vi "ArduinoRead.vi"(0 "VISA resource name":refnum<visa-resource-name>="COM24", 5 "Arduino function":enum16{"Interlock", "Edgesense", "Humidity"}(ring), 7 "Humidity IN":dbl[](array[numeric]), 9 "Temperature IN":dbl[](array[numeric]), 11 "error in (no error)":errorcluster) -> (2 "VISA resource name OUT":refnum<visa-resource-name>="COM24", 3 "Edgesense Status":u16(ring)=1 items=["Contact", "No contact"], 4 "Temperature [°C]":dbl, 6 "rel. Humidity [%]":dbl, 8 "Humidity OUT":dbl[](array[numeric]), 10 "Temperature OUT":dbl[](array[numeric]), 14 "error out":errorcluster, 15 "Interlock Status":u16(ring) items=["Dark", "Light"])   [LabVIEW 2013, in "ArduinoControl.lvclass"]
uses:
  ArduinoControl.lvclass
panel:
  out "String":string
  out "return count":u32
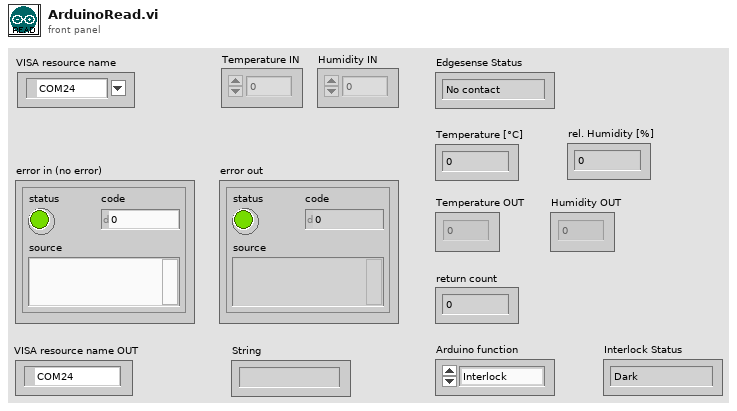
[diagram p1: front panel]
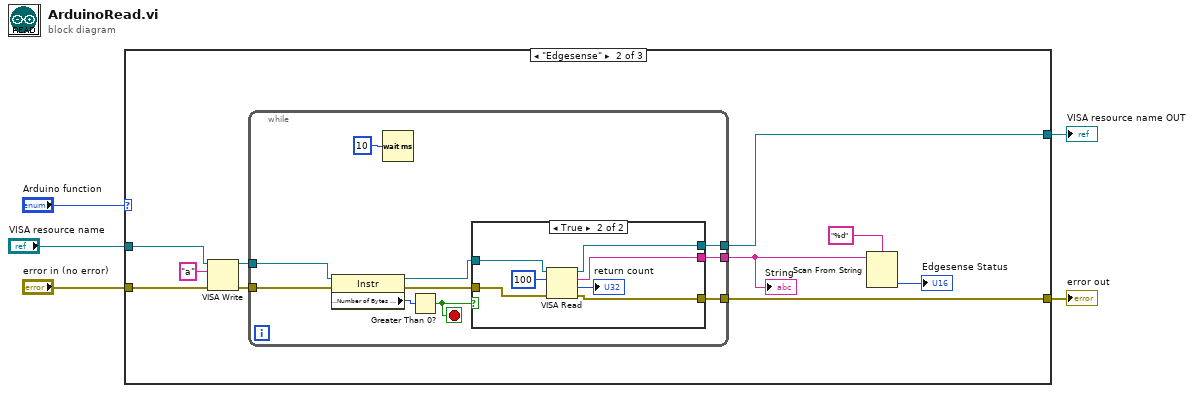
[diagram p0: block diagram]
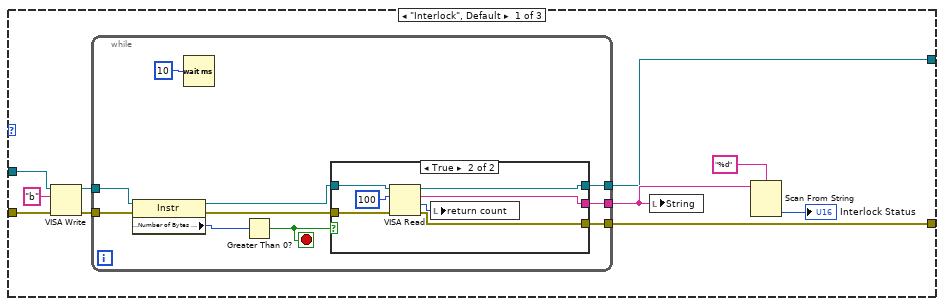
[diagram p2: hidden frame]
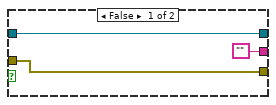
[diagram p3: hidden frame]
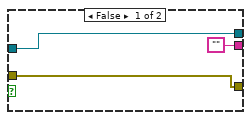
[diagram p4: hidden frame]
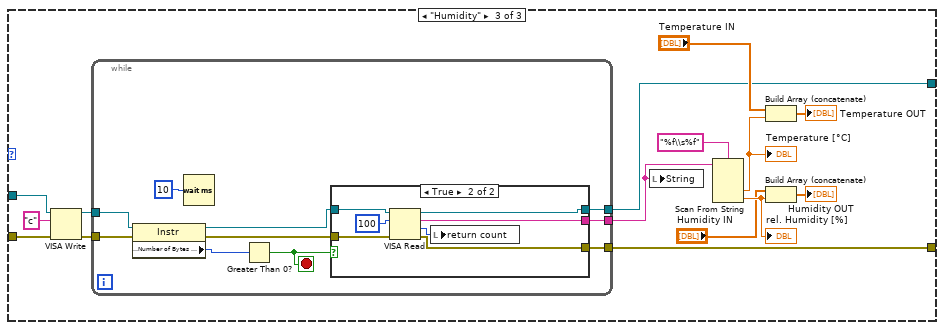
[diagram p5: hidden frame]
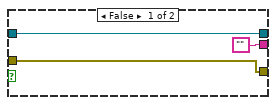
[diagram p6: hidden frame]
diagram:
  n1 = case shown="\"Edgesense\"" "Arduino function" {
    tunnel: "error in (no error)" -> [w7 w38 w68]
    tunnel: "VISA resource name" -> [w9 w39 w70]
    tunnel: [w12 w41 w71] -> w5
    tunnel: [w11 w42 w72] -> w4
    frame "Interlock", Default {
      n2 = VISA Write(VISA resource name=w9, write buffer="b", error in (no error)=w7) -> (VISA resource name out=w8:refnum<visa-resource-name>, error out=w6:errorcluster)  [unwired: 1 out]
      n3 = while {
        tunnel: [w23] -> w12
        tunnel: [w22] -> w13
        tunnel: w6 -> [w16]
        tunnel: w8 -> [w17]
        tunnel: [w21] -> w11
        stop <- w18 stop-if-true
        n4 = property class="Instr"(reference=w17, error in=w16) -> (reference out=w25:refnum<visa-resource-name>, error out=w24:errorcluster, "Serial Settings:Number of Bytes at Serial Port"=w19:u32)
        n5 = Wait (ms)(milliseconds to wait=10) -> ()  [unwired: 1 out]
        n6 = Greater Than 0?(x=w19) -> (x > 0?=w18:bool)
        n7 = case shown="True" w18 {
          tunnel: w25 -> [w26 w35]
          tunnel: w24 -> [w27 w34]
          tunnel: [w26 w33] -> w23
          tunnel: ["" w32] -> w22
          tunnel: [w27 w31] -> w21
          frame False {
          }
          frame True {
            n8 = VISA Read(VISA resource name=w35, byte count=100, error in (no error)=w34) -> (VISA resource name out=w33:refnum<visa-resource-name>, read buffer=w32:string, return count=w30:u32, error out=w31:errorcluster)
            n9 = local write "return count"(w30) -> ()
          }
        }
      }
      n10 = local write "String"(w13) -> ()
      n11 = Scan From String(format string="%d", input string=w13) -> (output 1=→"Interlock Status":u16)  [unwired: 3 in, 3 out]
    }
    frame "Edgesense" {
      n12 = VISA Write(VISA resource name=w39, write buffer="a", error in (no error)=w38) -> (VISA resource name out=w37:refnum<visa-resource-name>, error out=w36:errorcluster)  [unwired: 1 out]
      n13 = while {
        tunnel: [w53] -> w41
        tunnel: [w52] -> w43
        tunnel: w37 -> [w48]
        tunnel: [w51] -> w42
        tunnel: w36 -> [w49]
        stop <- w46 stop-if-true
        n14 = property class="Instr"(reference=w48, error in=w49) -> (reference out=w55:refnum<visa-resource-name>, error out=w54:errorcluster, "Serial Settings:Number of Bytes at Serial Port"=w47:u32)
        n15 = Wait (ms)(milliseconds to wait=10) -> ()  [unwired: 1 out]
        n16 = Greater Than 0?(x=w47) -> (x > 0?=w46:bool)
        n17 = case shown="True" w46 {
          tunnel: w55 -> [w56 w65]
          tunnel: w54 -> [w57 w64]
          tunnel: [w56 w63] -> w53
          tunnel: ["" w62] -> w52
          tunnel: [w57 w61] -> w51
          frame False {
          }
          frame True {
            n18 = VISA Read(VISA resource name=w65, byte count=100, error in (no error)=w64) -> (VISA resource name out=w63:refnum<visa-resource-name>, read buffer=w62:string, return count=→"return count":u32, error out=w61:errorcluster)
          }
        }
      }
      "String" <- w43
      n19 = Scan From String(format string="%d", input string=w43) -> (output 1=→"Edgesense Status":u16)  [unwired: 3 in, 3 out]
    }
    frame "Humidity" {
      n20 = VISA Write(VISA resource name=w70, write buffer="c", error in (no error)=w68) -> (VISA resource name out=w66:refnum<visa-resource-name>, error out=w67:errorcluster)  [unwired: 1 out]
      n21 = while {
        tunnel: [w88] -> w71
        tunnel: [w87] -> w73
        tunnel: w67 -> [w82]
        tunnel: w66 -> [w81]
        tunnel: [w86] -> w72
        stop <- w83 stop-if-true
        n22 = property class="Instr"(reference=w81, error in=w82) -> (reference out=w90:refnum<visa-resource-name>, error out=w89:errorcluster, "Serial Settings:Number of Bytes at Serial Port"=w84:u32)
        n23 = Wait (ms)(milliseconds to wait=10) -> ()  [unwired: 1 out]
        n24 = Greater Than 0?(x=w84) -> (x > 0?=w83:bool)
        n25 = case shown="True" w83 {
          tunnel: w90 -> [w91 w100]
          tunnel: w89 -> [w92 w99]
          tunnel: [w91 w98] -> w88
          tunnel: ["" w97] -> w87
          tunnel: [w92 w96] -> w86
          frame False {
          }
          frame True {
            n26 = VISA Read(VISA resource name=w100, byte count=100, error in (no error)=w99) -> (VISA resource name out=w98:refnum<visa-resource-name>, read buffer=w97:string, return count=w94:u32, error out=w96:errorcluster)
            n27 = local write "return count"(w94) -> ()
          }
        }
      }
      n28 = local write "String"(w73) -> ()
      n29 = Scan From String(format string="%f\\s%f", input string=w73) -> (output 1=w75:dbl, output 2=w80:dbl)  [unwired: 4 in, 3 out]
      "rel. Humidity [%]" <- w80
      "Temperature [°C]" <- w75
      n30 = Build Array (concatenate)("Temperature IN", w75) -> (→"Temperature OUT":dbl[])
      n31 = Build Array (concatenate)("Humidity IN", w80) -> (→"Humidity OUT":dbl[])
    }
  }
  "VISA resource name OUT" <- w5
  "error out" <- w4
